vi "get stats.vi"(8 "error in (no error)":errorcluster, 9 "Roy":u8[][](array[numeric]), 10 "Rob":u8[][](array[numeric]), 11 "Thorcam in":refnum<class "Thorcam.lvclass">) -> (0 "error out":errorcluster, 1 "Roy 2":u8[][](array[numeric]), 2 "Rob 2":u8[][](array[numeric]), 3 "Thorcam out":refnum<class "Thorcam.lvclass">)   [LabVIEW 2012]
uses:
  <vilib>/Analysis/NI_AALBase.lvlib
  Thorcam.lvclass
panel:
  in  "Rob":T1
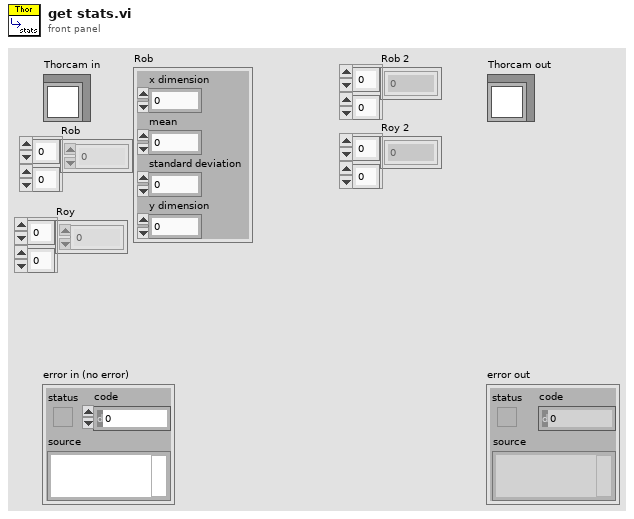
[diagram p1: front panel]
types:
  T1 = cluster{"x dimension":i32, "mean":dbl, "standard deviation":dbl, "y dimension":i32}
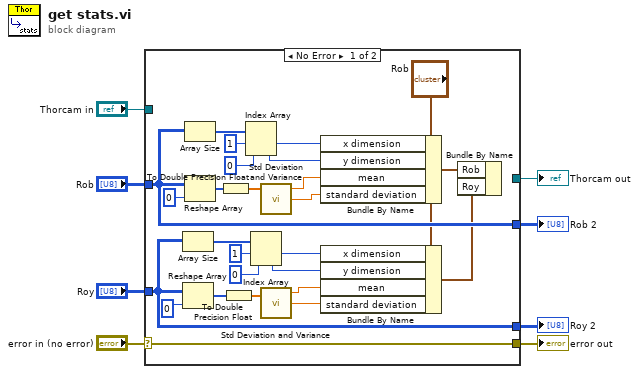
[diagram p0: block diagram]
diagram:
  n1 = case shown="No Error" "error in (no error)" {
    selector: "error in (no error)" -> [w34 w36]
    tunnel: [w34 w36] -> w7
    tunnel: [_ w35] -> w5
    tunnel: "Thorcam in" -> [_ w35]
    tunnel: "Rob" -> [w27 _]
    tunnel: "Roy" -> [w26 _]
    tunnel: [w26 _] -> w1
    tunnel: [w27 _] -> w2
    frame No Error {
      n2 = Array Size(array=w26) -> (size(s)=w20:i32[])
      n3 = Reshape Array(w26, 0 ("dimension size")) -> (w30:u8[])
      n4 = Array Size(array=w27) -> (size(s)=w25:i32[])
      n5 = Reshape Array(w27, 0 ("dimension size")) -> (w31:u8[])
      n6 = To Double Precision Float(number=w31) -> (double precision float=w33:dbl[])
      n7 = To Double Precision Float(number=w30) -> (double precision float=w32:dbl[])
      n8 = Index Array(array=w25, index #1=1 ("index"), index #2=0 ("index")) -> (element #1=w18:i32, element #2=w17:i32)
      n9 = Index Array(array=w20, index #1=1 ("index"), index #2=0 ("index")) -> (element #1=w14:i32, element #2=w13:i32)
      n10 = call <vilib>:"Std Deviation and Variance.vi"("X"=w33) -> ("mean"=w16:dbl, "standard deviation"=w15:dbl)  [unwired: 1 in, 1 out]
      n11 = call <vilib>:"Std Deviation and Variance.vi"("X"=w32) -> ("mean"=w12:dbl, "standard deviation"=w11:dbl)  [unwired: 1 in, 1 out]
      n12 = Bundle By Name(cluster="Rob", "x dimension"=w18, "y dimension"=w17, "mean"=w16, "standard deviation"=w15) -> (w19:T1)
      n13 = Bundle By Name(cluster="Rob", "x dimension"=w14, "y dimension"=w13, "mean"=w12, "standard deviation"=w11) -> (w9:T1)
      n14 = Bundle By Name("Rob"=w19, "Roy"=w9) -> ()  [unwired: 1 in, 1 out]
    }
    frame Error {
    }
  }
  "error out" <- w7
  "Thorcam out" <- w5
  "Rob 2" <- w2
  "Roy 2" <- w1
